vi "test_organizar_tags.vi"() -> ()   [LabVIEW 2015]
uses:
  Library/IF2_Reader/IF2_Reader.lvlib
panel:
  out "Array 6":string[](array[string])
  out "upper_limit 2":u64
  out "tag time 2":u64
  out "Array 5":string[][](array[string])
  out "Array 4":u64[][](array[numeric])
  out "Array 3":u64[][](array[numeric])
  out "Array 2":u64[][](array[numeric])
  out "Array":bool[](array[boolean])
  out "x*y":dbl
  out "tag time":u64
  out "lower_limit":u64
  out "upper_limit":u64
  out "FirstSeemUs":u64
  in  "Tabla_flota":string[][](array[string])=[["Flota", "UT", "Ejes", "Tag inicio", "Tag fin"], ["Prueba", "1", "4", "A0000000000000000TESTNEM7", "A0000000000000000TESTNEM8"], ["Riyadh Metro L3", "Train01", "8", "200917000000000000001196", "200917000000000000001195"], ["Riyadh Metro L3", "Train02", "8", "200917000000000000001277", "200917000000000000001293"], ["Riyadh Metro L3", "Train03", "8", "2009170000000000000012B7", "200917000000000000001259"], ["Riyadh Metro L3", "Train04", "8", "2009170000000000000011B3", "20091700000000000000119F"], ["Riyadh Metro L3", "Train05", "8", "2009170000000000000012E6", "2009170000000000000012AF"], ["Riyadh Metro L3", "Train06", "8", "200917000000000000001227", "2009170000000000000012B9"], ["Riyadh Metro L3", "Train07", "8", "200917000000000000001272", "2009170000000000000011FA"], ["Riyadh Metro L3", "Train08", "8", "200917000000000000001225", "2009170000000000000012BC"], ["Riyadh Metro L3", "Train09", "8", "200917000000000000001226", "2009170000000000000011C8"], ["Riyadh Metro L3", "Train10", "8", "2009170000000000000011FC", "2009170000000000000012B8"], ["Riyadh Metro L3", "Train11", "8", "200917000000000000001197", "20091700000000000000124C"], ["Riyadh Metro L3", "Train12", "8", "20091700000000000000124F", "2009170000000000000011BF"], ["Riyadh Metro L3", "Train13", "8", "2009170000000000000011CA", "200917000000000000001198"], ["Riyadh Metro L3", "Train14", "8", "2009170000000000000011DA", "2009170000000000000011D9"], ["Riyadh Metro L3", "Train15", "8", "20091700000000000000121C", "20091700000000000000122C"], ["Riyadh Metro L3", "Train16", "8", "2009170000000000000011B9", "200917000000000000001214"], ["Riyadh Metro L3", "Train17", "8", "200917000000000000001222", "2009170000000000000011B6"], ["Riyadh Metro L3", "Train18", "8", "200917000000000000001229", "200917000000000000001200"], ["Riyadh Metro L3", "Train19", "8", "200917000000000000001217", "200917000000000000001232"], ["Riyadh Metro L3", "Train20", "8", "2009170000000000000012B4", "2009170000000000000011CE"], ["Riyadh Metro L3", "Train21", "8", "2009170000000000000011A8", "2009170000000000000011F6"], ["Riyadh Metro L3", "Train22", "8", "200917000000000000001220", "2009170000000000000011C4"], ["Riyadh Metro L3", "Train23", "8", "2009170000000000000011EA", "200917000000000000001208"], ["Riyadh Metro L3", "Train24", "8", "200917000000000000001219", "20091700000000000000121A"], ["Riyadh Metro L3", "Train25", "8", "200917000000000000001348", "2009170000000000000012B2"], ["Riyadh Metro L3", "Train26", "8", "2009170000000000000011BD", "2009170000000000000011F7"], ["Riyadh Metro L3", "Train27", "8", "200917000000000000001207", "200917000000000000001206"], ["Riyadh Metro L3", "Train28", "8", "200917000000000000001230", "200917000000000000001322"], ["Riyadh Metro L3", "Train29", "8", "2009170000000000000011BE", "20091700000000000000124B"], ["Riyadh Metro L3", "Train30", "8", "2009170000000000000011E2", "2009170000000000000011A7"], ["Riyadh Metro L3", "Train31", "8", "2009170000000000000012BE", "2009170000000000000012BD"], ["Riyadh Metro L3", "Train32", "8", "2009170000000000000012B6", "200917000000000000001323"], ["Riyadh Metro L3", "Train33", "8", "200917000000000000001216", "20091700000000000000122A"], ["Riyadh Metro L3", "Train34", "8", "200917000000000000001274", "200917000000000000001291"], ["Riyadh Metro L3", "Train35", "8", "2009170000000000000012C4", "200917000000000000001253"], ["Riyadh Metro L3", "Train36", "8", "2009170000000000000011BC", "200917000000000000001228"], ["Riyadh Metro L3", "Train37", "8", "200917000000000000001205", "200917000000000000001292"], ["Riyadh Metro L3", "Train38", "8", "2009170000000000000011FF", "2009170000000000000011AA"], ["Riyadh Metro L3", "Train39", "8", "2009170000000000000012C5", "200917000000000000001223"], ["Riyadh Metro L3", "Train40", "8", "200917000000000000001231", "200917000000000000001199"], ["Riyadh Metro L3", "Train41", "8", "2009170000000000000011C7", "20091700000000000000121F"], ["Riyadh Metro L3", "Train42", "8", "2009170000000000000011AC", "2009170000000000000011AB"], ["Riyadh Metro L3", "Train43", "8", "20091700000000000000121D", "200917000000000000001302"], ["Riyadh Metro L3", "Train44", "8", "2009170000000000000011CD", "2009170000000000000011E1"], ["Riyadh Metro L3", "Train45", "8", "2009170000000000000012B0", "2009170000000000000011A0"], ["Riyadh Metro L3", "Train46", "8", "2009170000000000000012BB", "2009170000000000000012BA"], ["Riyadh Metro L3", "Train47", "8", "20091700000000000000119C", "20091700000000000000119B"], ["test Tag", "Train48", "8", "200917000000000000000184", "200917000000000000000183"]]
  in  "Inicio pasada 2":timestamp=timestamp(3739428458.436 s since 1904-01-01)
  out "unixTimeStamp":u64
  out "double precision float":u64
  in  "Inicio pasada":timestamp=timestamp(3739428458.436 s since 1904-01-01)
  in  "TagData in":cluster{"TagCode":string, "FirstSeemUs":u64}[](array[cluster])
  in  "Tiempo de paso (s)":dbl
  out "Tags":string[](array[string])
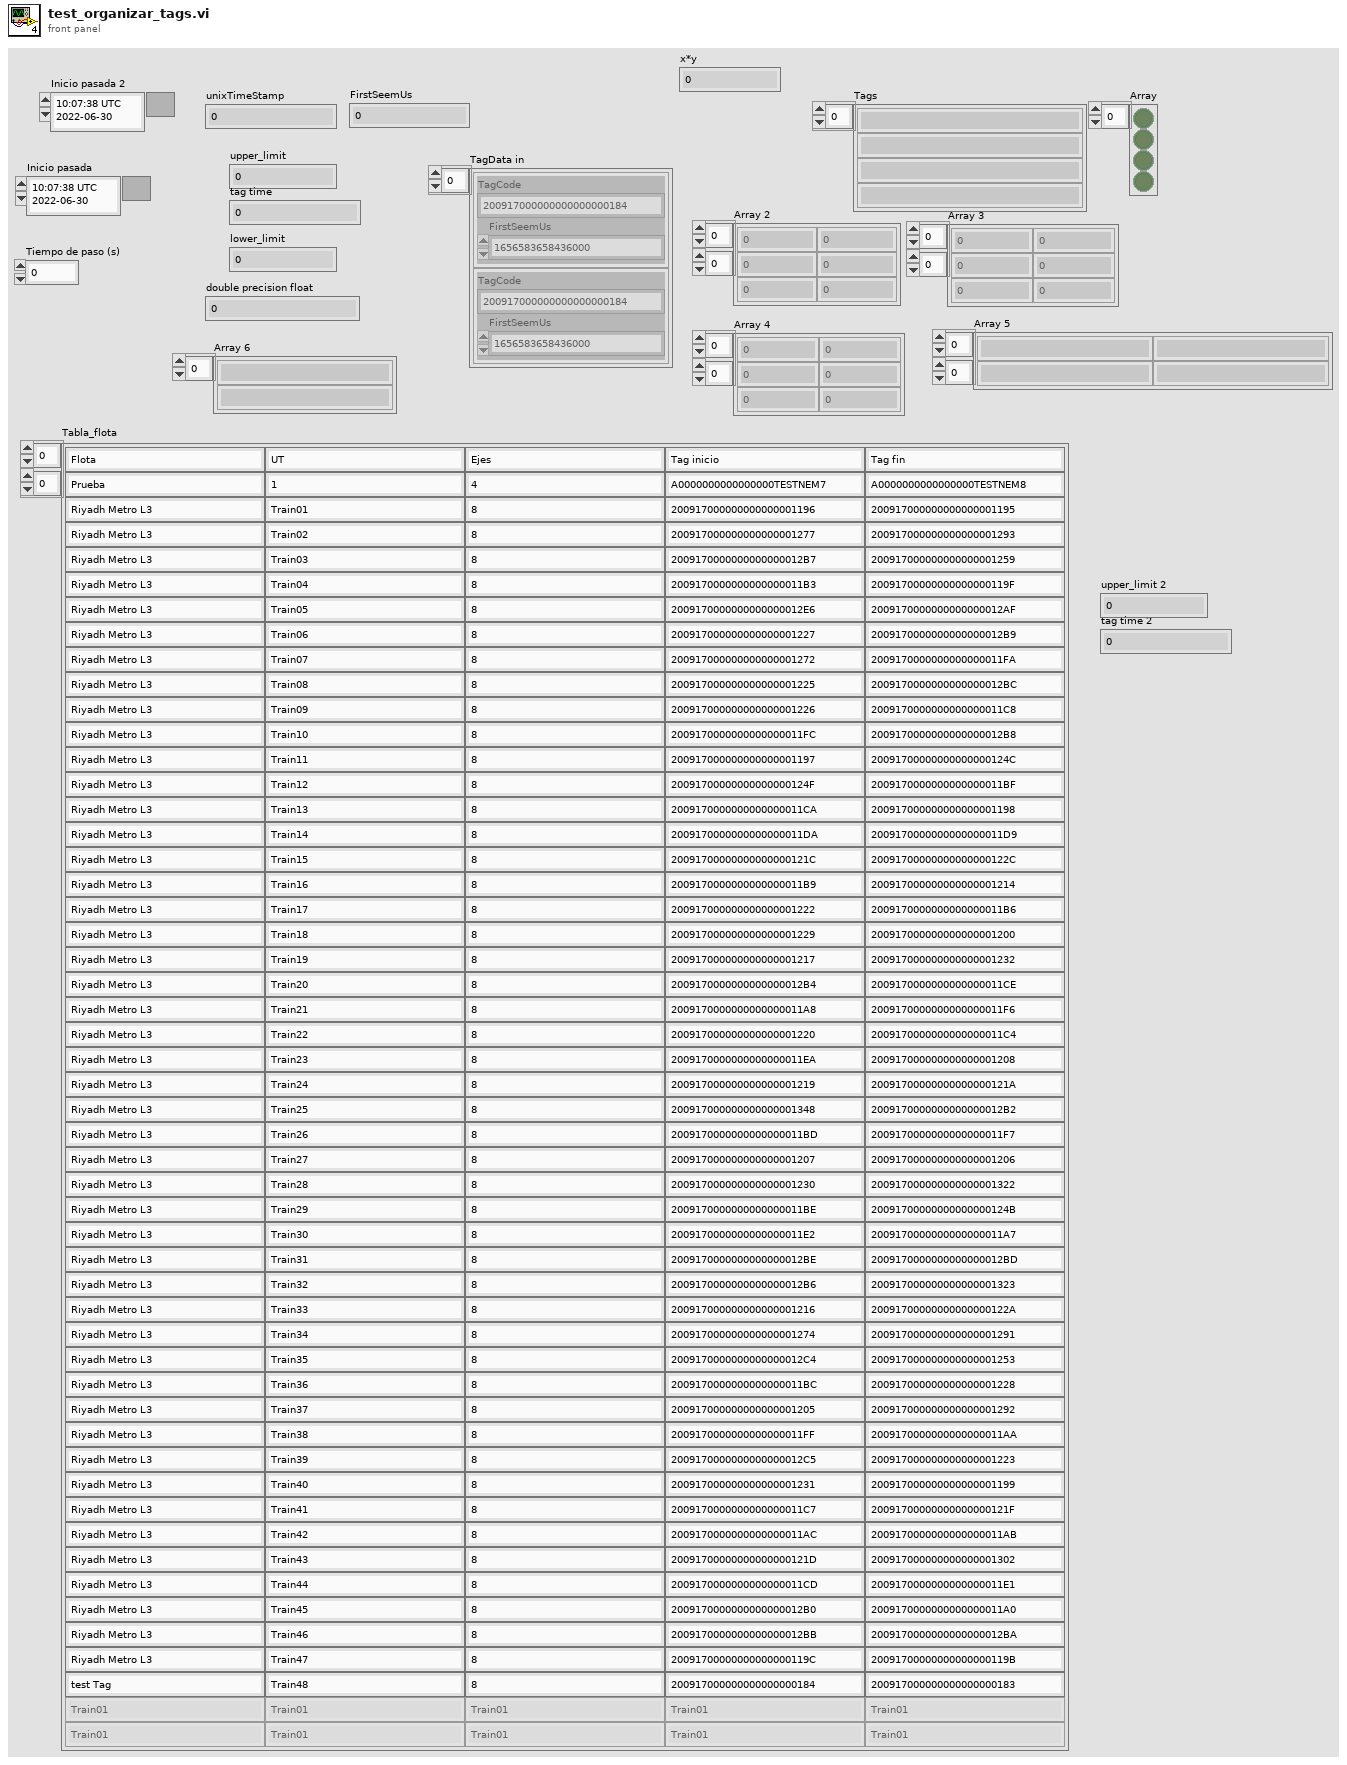
[diagram p1: front panel]
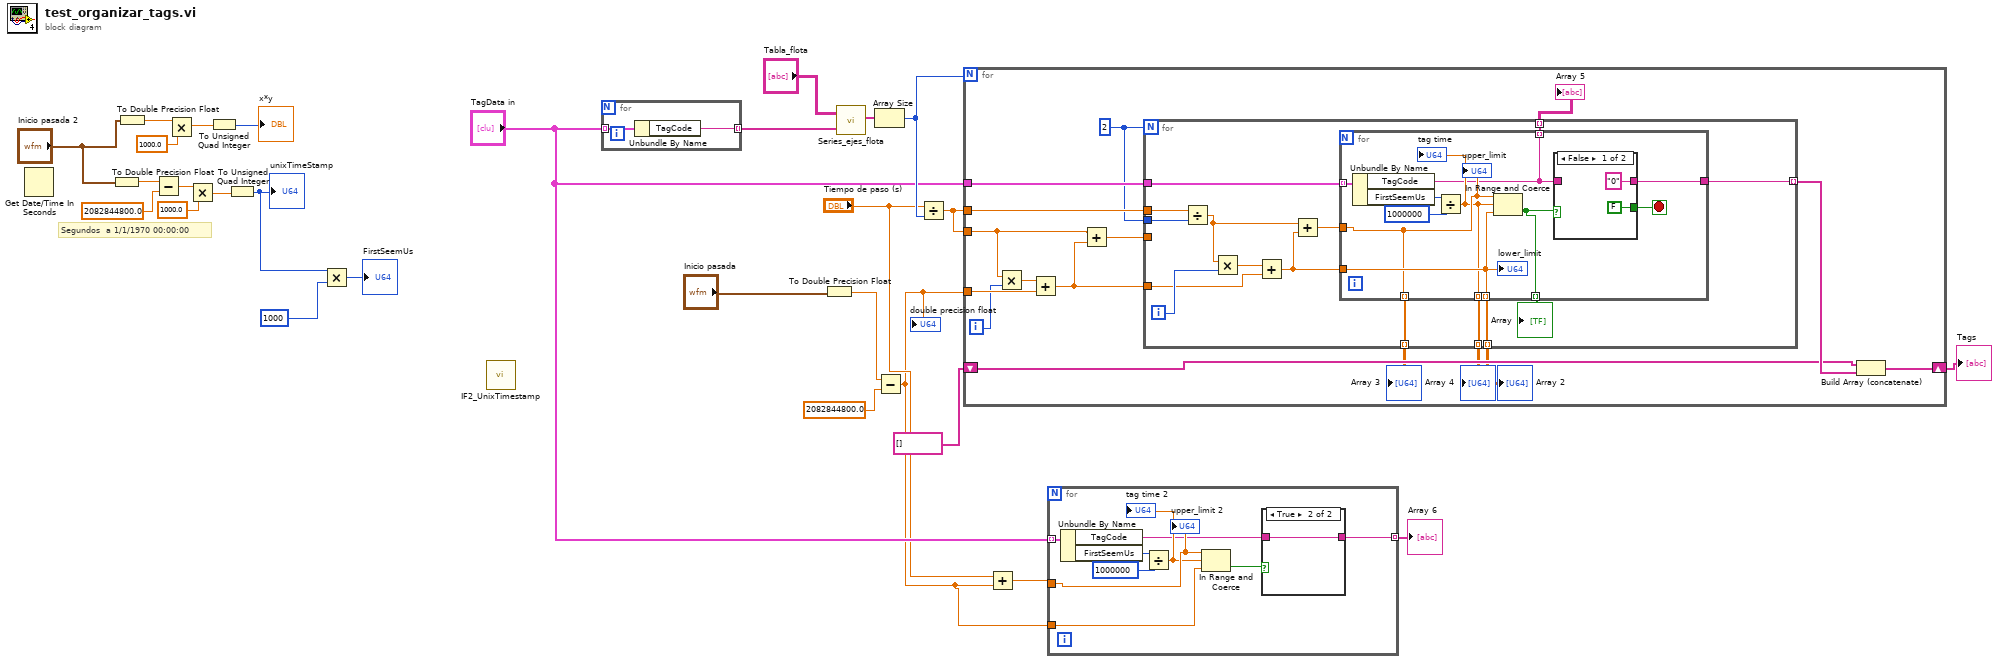
[diagram p0: block diagram]
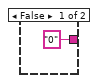
[diagram p2: hidden frame]
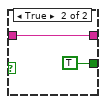
[diagram p3: hidden frame]
diagram:
  # "Segundos  a 1/1/1970 00:00:00"
  n1 = Get Date/Time In Seconds() -> ()  [unwired: 1 out]
  n2 = To Double Precision Float(number="Inicio pasada 2") -> (double precision float=w25:dbl)
  n3 = To Double Precision Float(number="Inicio pasada 2") -> (double precision float=w10:dbl)
  n4 = Subtract(x=w25, y=2082844800.0) -> (x-y=w26:dbl)
  n5 = Multiply(x=w10, y=1000.0) -> (x*y=w9:dbl)
  n6 = Multiply(x=w26, y=1000.0) -> (x*y=w28:dbl)
  n7 = To Unsigned Quad Integer(1:w9) -> (0:→"x*y":u64)
  n8 = To Unsigned Quad Integer(1:w28) -> (0:w23:u64)
  "unixTimeStamp" <- w23
  n9 = Multiply(x=w23, y=u64 1000) -> (x*y=→"FirstSeemUs":u64)
  n10 = call "IF2_UnixTimestamp.vi"() -> ()  [unwired: 11 in, 1 out]
  n11 = for {
    tunnel: "TagData in" -> [w30] mode=indexing
    tunnel: [w29] -> w19 mode=indexing
    n12 = Unbundle By Name(w30) -> ("TagCode"=w29:string)
  }
  n13 = To Double Precision Float(number="Inicio pasada") -> (double precision float=w6:dbl)
  n14 = call "Series_ejes_flota.vi"("Tabla_flota"="Tabla_flota", "Tags"=w19) -> ("Series del convoy"=w18:string[])  [unwired: 2 in, 2 out]
  n15 = Array Size(array=w18) -> (size(s)=w20:i32)
  n16 = Subtract(x=w6, y=2082844800.0) -> (x-y=w2:dbl)
  "double precision float" <- w2
  n17 = Divide(x="Tiempo de paso (s)", y=w20) -> (x/y=w21:dbl)
  n18 = for {
    N: w20 -> [_]
    tunnel: w2 -> [w45]
    tunnel: w21 -> [w44]
    tunnel: "TagData in" -> [w43]
    tunnel: w21 -> [w40]
    shift-right: [w37] -> w16
    shift-left: string[] [] -> [w36]
    i -> [w35]
    w39 = 2
    n19 = Multiply(x=w44, y=w35) -> (x*y=w46:dbl)
    n20 = Add(x=w46, y=w45) -> (x+y=w41:dbl)
    n21 = Add(x=w44, y=w41) -> (x+y=w42:dbl)
    n22 = for {
      N: w39 -> [_]
      tunnel: w43 -> [w61]
      tunnel: w42 -> [_]
      tunnel: w41 -> [w56]
      tunnel: w40 -> [w60]
      tunnel: w39 -> [w59]
      tunnel: [w52] -> w38 mode=indexing
      tunnel: [w50] -> w34 mode=indexing
      tunnel: [w49] -> w33 mode=indexing
      tunnel: [w48] -> w32 mode=indexing
      tunnel: [w47] -> w31 mode=indexing
      i -> [w58]
      n23 = Divide(x=w60, y=w59) -> (x/y=w54:dbl)
      n24 = Multiply(x=w54, y=w58) -> (x*y=w57:dbl)
      n25 = Add(x=w57, y=w56) -> (x+y=w55:dbl)
      n26 = Add(x=w54, y=w55) -> (x+y=w53:dbl)
      n27 = for {
        tunnel: w61 -> [w71] mode=indexing
        tunnel: w55 -> [w66]
        tunnel: w53 -> [w65]
        tunnel: [w68] -> w52
        tunnel: [w67] -> w51 mode=indexing
        tunnel: [w66] -> w50 mode=indexing
        tunnel: [w65] -> w49 mode=indexing
        tunnel: [w64] -> w48 mode=indexing
        tunnel: [w63] -> w47 mode=indexing
        stop <- w62 stop-if-true
        n28 = Unbundle By Name(w71) -> ("TagCode"=w63:string, "FirstSeemUs"=w70:u64)
        n29 = Divide(x=w70, y=u64 1000000) -> (x/y=w64:dbl)
        "tag time" <- w64
        n30 = In Range and Coerce(upper limit=w65, x=w64, lower limit=w66) -> (In Range?=w67:bool)  [unwired: 1 out]
        n31 = case shown="False" w67 {
          tunnel: w63 -> [_ w75]
          tunnel: ["0" ("TagCode") w75] -> w68
          tunnel: [FALSE TRUE] -> w62
          frame False {
          }
          frame True {
          }
        }
        "upper_limit" <- w65
        "lower_limit" <- w66
      }
      "Array" <- w51
    }
    "Array 2" <- w34
    "Array 3" <- w33
    "Array 4" <- w32
    "Array 5" <- w31
    n32 = Build Array (concatenate)(w36, w38) -> (w37:string[])
  }
  "Tags" <- w16
  n33 = Add(x="Tiempo de paso (s)", y=w2) -> (x+y=w4:dbl)
  n34 = for {
    tunnel: "TagData in" -> [w84] mode=indexing
    tunnel: w2 -> [w81]
    tunnel: w4 -> [w80]
    tunnel: [w76] -> w1 mode=indexing
    n35 = Unbundle By Name(w84) -> ("TagCode"=w78:string, "FirstSeemUs"=w83:u64)
    n36 = Divide(x=w83, y=u64 1000000) -> (x/y=w79:dbl)
    "tag time 2" <- w79
    n37 = In Range and Coerce(upper limit=w80, x=w79, lower limit=w81) -> (In Range?=w77:bool)  [unwired: 1 out]
    n38 = case shown="True" w77 {
      tunnel: w78 -> [_ w86]
      tunnel: ["0" ("TagCode") w86] -> w76
      frame False {
      }
      frame True {
      }
    }
    "upper_limit 2" <- w80
  }
  "Array 6" <- w1
